vi "BatchProcess-111.vi"() -> ()   [LabVIEW 2015]
uses:
  CustomVIs/CustomVI.lvlib
panel:
  out "element 2":string
  out "output 2":timestamp
  out "element":string
  out "output 1":timestamp
  in  "Path":path
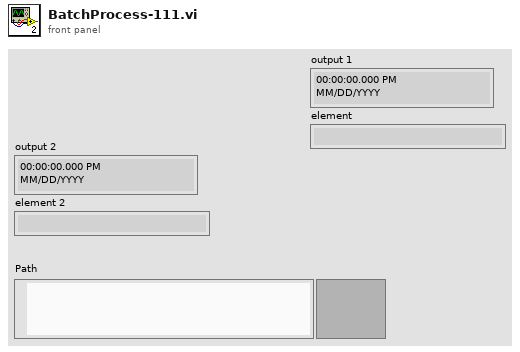
[diagram p1: front panel]
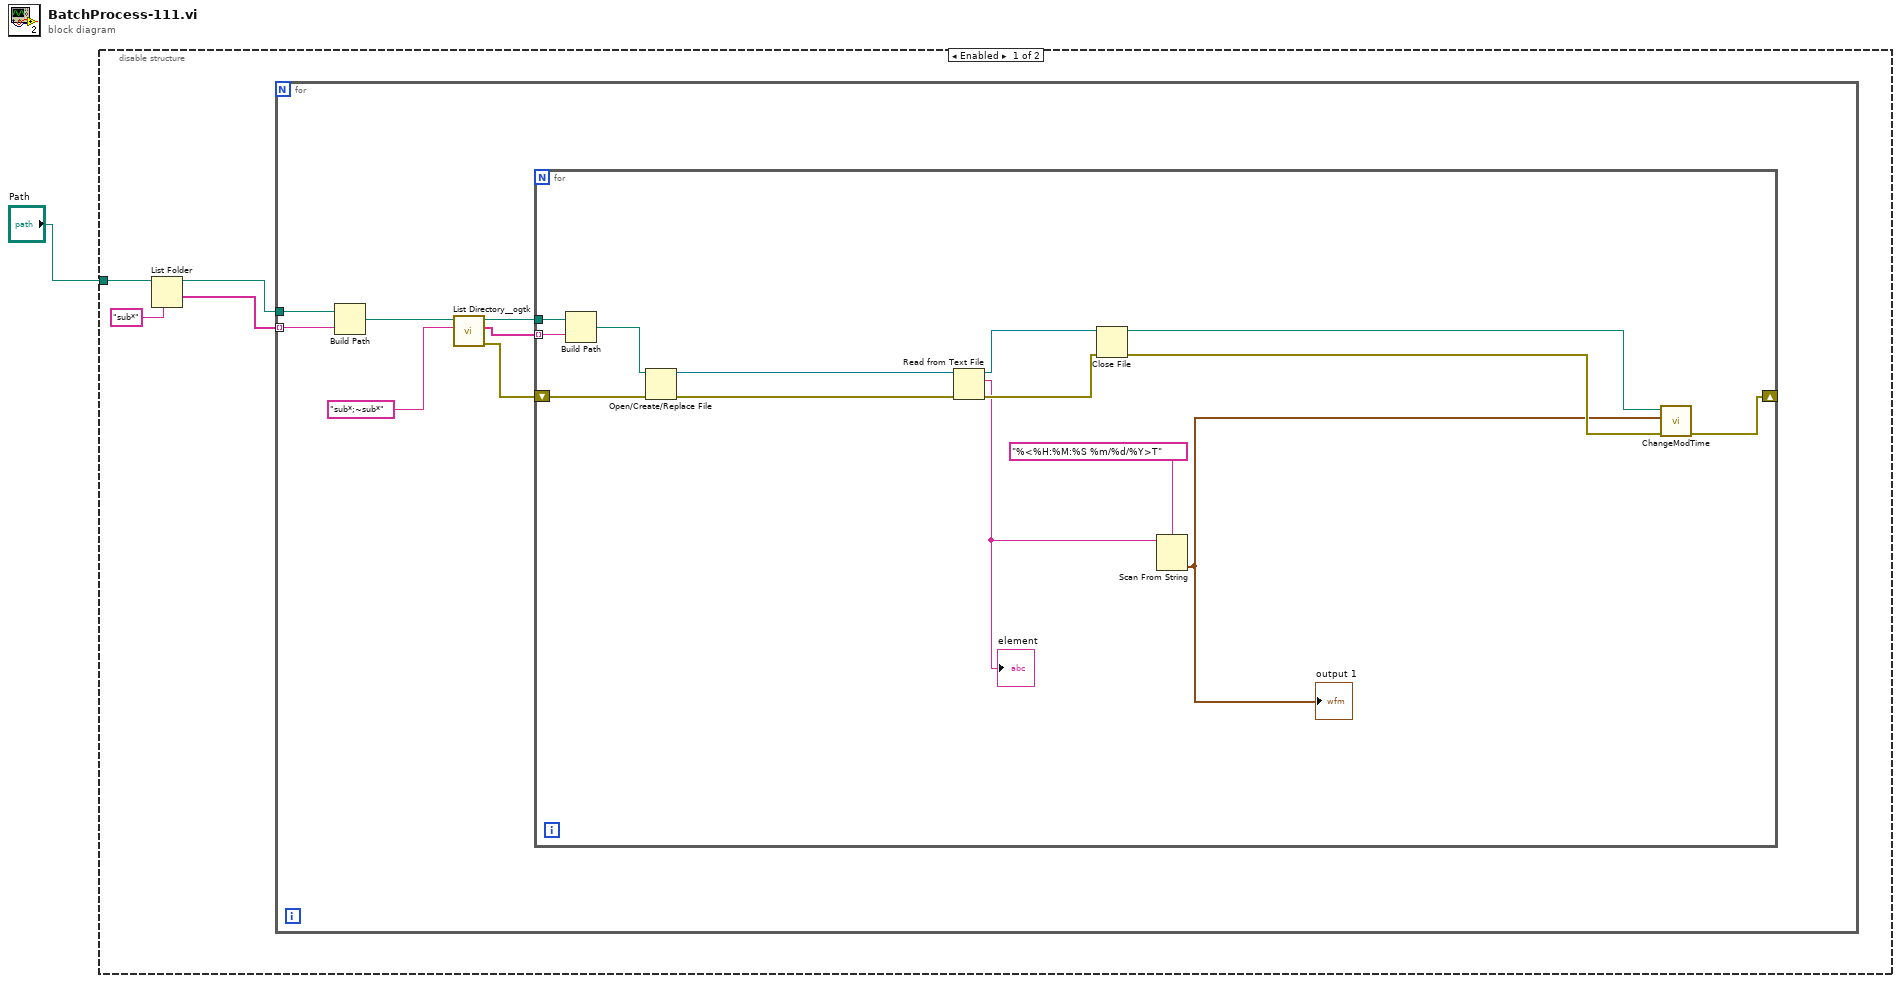
[diagram p0: block diagram]
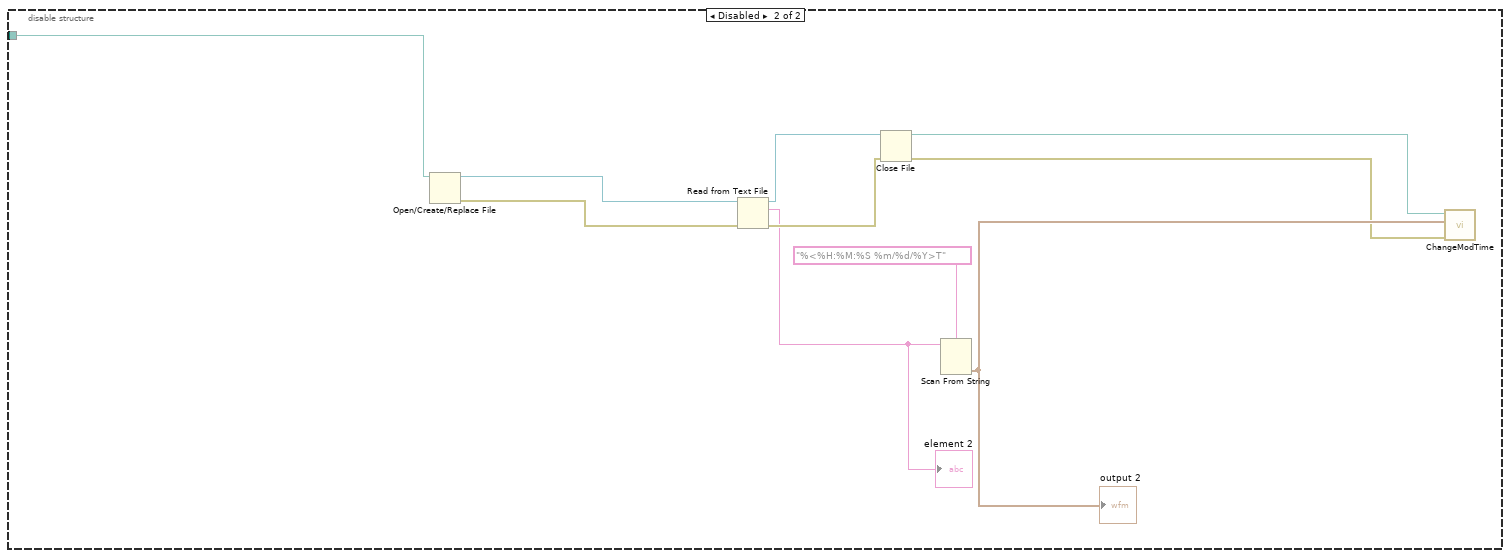
[diagram p2: hidden frame]
diagram:
  n1 = disable-structure shown="Enabled" {
    disable-tunnel: "Path" -> [w5 w28]
    frame Enabled {
      n2 = List Folder(path=w5, pattern="sub*") -> (path out=w4:path, folder names=w3:string[])  [unwired: 2 in, 2 out]
      n3 = for {
        tunnel: w4 -> [w9]
        tunnel: w3 -> [w7] mode=indexing
        n4 = Build Path(base path=w9, name or relative path=w7) -> (appended path=w8:path)
        n5 = call <userlib>:"List Directory__ogtk.vi"("pattern"="sub*;~sub*", "directory path"=w8) -> ("error out"=w10:errorcluster, "file names"=w11:string[], "dup directory path"=w12:path)  [unwired: 2 in, 1 out]
        n6 = for {
          tunnel: w12 -> [w19]
          tunnel: w11 -> [w20] mode=indexing
          shift-right: [w16] -> _
          shift-left: w10 -> [w17]
          n7 = Build Path(base path=w19, name or relative path=w20) -> (appended path=w18:path)
          n8 = Open/Create/Replace File(file path (use dialog)=w18, error in=w17) -> (refnum out=w15:refnum<file>, error out=w14:errorcluster)  [unwired: 4 in, 1 out]
          n9 = Read from Text File(file (use dialog)=w15, error in=w14) -> (refnum out=w25:refnum<file>, text=w13:string, error out=w26:errorcluster)  [unwired: 2 in, 1 out]
          "element" <- w13
          n10 = Close File(refnum=w25, error in=w26) -> (path=w23:path, error out=w24:errorcluster)
          n11 = Scan From String(format string="%<%H:%M:%S %m/%d/%Y>T", input string=w13) -> (output 1=w21:timestamp)  [unwired: 3 in, 3 out]
          "output 1" <- w21
          n12 = call "ChangeModTime.vi"("error in (no error)"=w24, "Time Stamp"=w21, "path"=w23) -> ("error out"=w16:errorcluster)  [unwired: 7 in, 1 out]
        }
      }
    }
    frame Disabled {
      n13 = Open/Create/Replace File(file path (use dialog)=w28) -> (refnum out=w35:refnum<file>, error out=w36:errorcluster)  [unwired: 5 in, 1 out]
      n14 = Read from Text File(file (use dialog)=w35, error in=w36) -> (refnum out=w30:refnum<file>, text=w27:string, error out=w29:errorcluster)  [unwired: 2 in, 1 out]
      "element 2" <- w27
      n15 = Close File(refnum=w30, error in=w29) -> (path=w32:path, error out=w31:errorcluster)
      n16 = Scan From String(format string="%<%H:%M:%S %m/%d/%Y>T", input string=w27) -> (output 1=w34:timestamp)  [unwired: 3 in, 3 out]
      "output 2" <- w34
      n17 = call "ChangeModTime.vi"("error in (no error)"=w31, "Time Stamp"=w34, "path"=w32) -> ()  [unwired: 7 in, 2 out]
    }
  }
